vi "Configure Mask Test.vi"   [LabVIEW 2010, in "Agilent 2000 3000 X-Series.lvlib"]
doc: "Configures the setttings of mast test."
uses:
  <instrlib>/Agilent 2000 3000 X-Series/Agilent 2000 3000 X-Series.lvlib
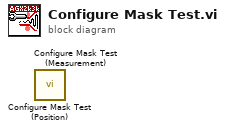
[diagram p0: block diagram]
diagram:
  n1 = call <instrlib>:"Configure Mask Test (Position).vi"() -> ()  [unwired: 14 in, 2 out]
  n2 = call <instrlib>:"Configure Mask Test (Measurement).vi"() -> ()  [unwired: 14 in, 2 out]
